vi "Assert Channel Configurations Match.vi"(8 "error in (no error)":errorcluster, 9 "Channel Configurations":T5(array[cluster]), 10 "Channel Refs":T1[](array[typedef]) format="%.0x", 11 "Test Case in":refnum<class "Routing and Faulting Import Unit Tests.lvclass">) -> (0 "error out":errorcluster, 3 "Test Case out":refnum<class "Routing and Faulting Import Unit Tests.lvclass">)   [LabVIEW 2020, in "Routing and Faulting Import Unit Tests.lvclass"]
uses:
  Routing and Faulting Import Unit Tests.lvclass
  Shared/Channel States.ctl
  Shared/Routing State.ctl
  Shared/Connection.ctl
  <vilib>/NI VeriStand/Custom Device API/Custom Device Item Ref.ctl
  Scripting/Routing and Faulting Scripting.lvlib
  Shared/Routing and Faulting Shared.lvlib
  <vilib>/NI VeriStand/Custom Device API/Custom Device API.lvlib
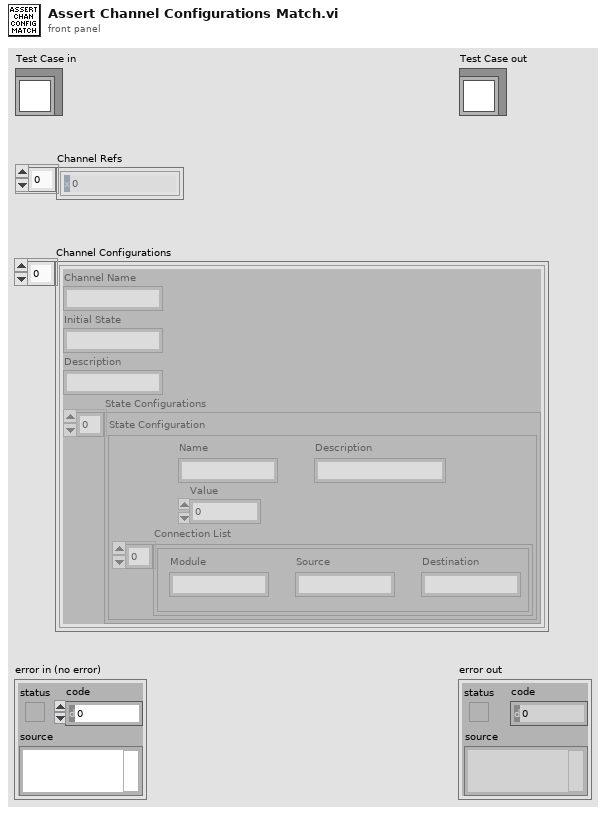
[diagram p1: front panel]
types:
  T1 = typedef "Custom Device API.lvlib/Custom Device Item Ref.ctl" = u64
  T2 = typedef "Routing and Faulting Shared.lvlib/Channel States.ctl" = T3[]
  T3 = typedef "Routing and Faulting Shared.lvlib/Routing State.ctl" = cluster{"Name":string, "Description":string, "Value":i32, "Connection List":T4[]}
  T4 = typedef "Routing and Faulting Shared.lvlib/Connection.ctl" = cluster{"Module":string, "Source":string, "Destination":string}
  T5 = cluster{"Channel Name":string, "Initial State":string, "Description":string, "State Configurations":T2}[]
  T6 = cluster{"Channel Name":string, "Initial State":string, "Description":string, "State Configurations":T2}
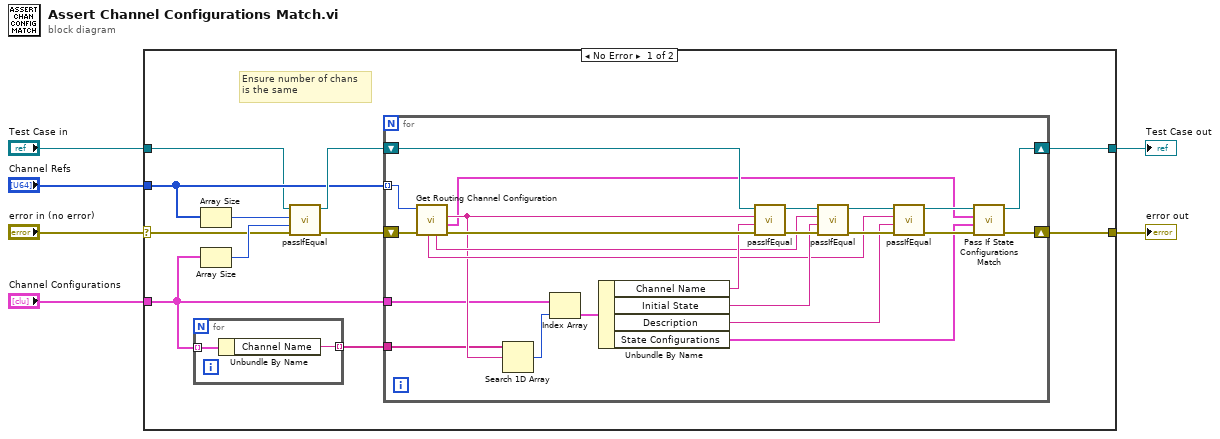
[diagram p0: block diagram]
diagram:
  n1 = case shown="No Error" "error in (no error)" {
    selector: "error in (no error)" -> [w10 w45]
    tunnel: [w7 w45] -> w5
    tunnel: [w8 w44] -> w3
    tunnel: "Test Case in" -> [w9 w44]
    tunnel: "Channel Configurations" -> [w11 _]
    tunnel: "Channel Refs" -> [w12 _]
    frame No Error {
      # "Ensure number of chans\nis the same"
      n2 = for {
        tunnel: [w19] -> w17 mode=indexing
        tunnel: w11 -> [w18] mode=indexing
        n3 = Unbundle By Name(w18) -> ("Channel Name"=w19:string)
      }
      n4 = Array Size(array=w12) -> (size(s)=w14:i32)
      n5 = Array Size(array=w11) -> (size(s)=w13:i32)
      n6 = call-dynamic "passIfEqual.vi"("error in (no error)"=w10, "y"=w13, "x"=w14, "TestCase in"=w9) -> ("error out"=w16:errorcluster, "TestCase out"=w15:refnum<class "Routing and Faulting Import Unit Tests.lvclass">)  [unwired: 6 in]
      n7 = for {
        tunnel: w12 -> [w42] mode=indexing
        shift-right: [w20] -> w8
        shift-left: w15 -> [w40]
        shift-right: [w24] -> w7
        shift-left: w16 -> [w43]
        tunnel: w11 -> [w28]
        tunnel: w17 -> [w27]
        n8 = call "Get Routing Channel Configuration.vi"("error in"=w43, "routing channel in"=w42) -> ("error out"=w41:errorcluster, "state configurations"=w22:T2, "routing channel name"=w30:string, "initial state"=w34:string, "description"=w32:string)  [unwired: 4 in, 1 out]
        n9 = Search 1D Array(1D array=w27, element=w30) -> (index of element=w26:i32)  [unwired: 1 in]
        n10 = Index Array(array=w28, index=w26) -> (element=w29:T6)
        n11 = Unbundle By Name(w29) -> ("Channel Name"=w35:string, "Initial State"=w33:string, "Description"=w31:string, "State Configurations"=w21:T2)
        n12 = call-dynamic "passIfEqual.vi"("error in (no error)"=w41, "y"=w35, "x"=w30, "TestCase in"=w40) -> ("error out"=w39:errorcluster, "TestCase out"=w37:refnum<class "Routing and Faulting Import Unit Tests.lvclass">)  [unwired: 6 in]
        n13 = call-dynamic "passIfEqual.vi"("error in (no error)"=w39, "y"=w33, "x"=w34, "TestCase in"=w37) -> ("error out"=w38:errorcluster, "TestCase out"=w36:refnum<class "Routing and Faulting Import Unit Tests.lvclass">)  [unwired: 6 in]
        n14 = call-dynamic "passIfEqual.vi"("error in (no error)"=w38, "y"=w31, "x"=w32, "TestCase in"=w36) -> ("error out"=w25:errorcluster, "TestCase out"=w23:refnum<class "Routing and Faulting Import Unit Tests.lvclass">)  [unwired: 6 in]
        n15 = call "Pass If State Configurations Match.vi"("error in (no error)"=w25, "Known State Configurations"=w21, "Imported State Configurations"=w22, "Test Case in"=w23) -> ("error out"=w24:errorcluster, "Test Case out"=w20:refnum<class "Routing and Faulting Import Unit Tests.lvclass">)  [unwired: 6 in]
      }
    }
    frame Error {
    }
  }
  "error out" <- w5
  "Test Case out" <- w3
